vi "Glowy_Projekt.vi"() -> ()   [LabVIEW 2023]
uses:
  <vilib>/Utility/miscctls.llb/LVDateTimeRec.ctl
  stan.ctl
  Zmienn_globalne.vi
  Ogrod_zmienne.vi
  Rosliny_zmienne.vi
  Trawnik_zmienne.vi
panel:
  out "Wilgotnosc":dbl(slide)=50.0 scale=0.0..100.0
  out "Naslonecznienie":dbl(slide) scale=0.0..100.0
  in  "Przyspieszenie czasu":dbl(knob)=1.0 scale=1.0..2000.0
  out "Czas podlewania reczny":dbl
  out "date time rec":T1
  in  "Oproznianie":dbl(slide) scale=0.0..1.0
  in  "Intensywnosc opadow":dbl(slide) scale=0.0..1.0
  out "Zbiornik retencyjny":dbl(slide)=50.0 scale=0.0..100.0
  out "Aktywne podlewanie rabat roslinnych":bool
  out "Aktywne podlewanie warzywniak":bool
  out "Aktywne podlewanie sekcja 5":bool
  out "Aktywne podlewanie sekcja 4":bool
  out "Aktywne podlewanie sekcja 3":bool
  out "Aktywne podlewanie sekcja 2":bool
  out "Aktywne podlewanie sekcja 1":bool
  in  "Rosliny":bool
  in  "Ogród Warzywny":bool
  in  "Trawnik":bool
  out "Numeric":i32
  # "Trawnik"
  # "Warzywniak"
  # "DOM"
  # "Rosliny"
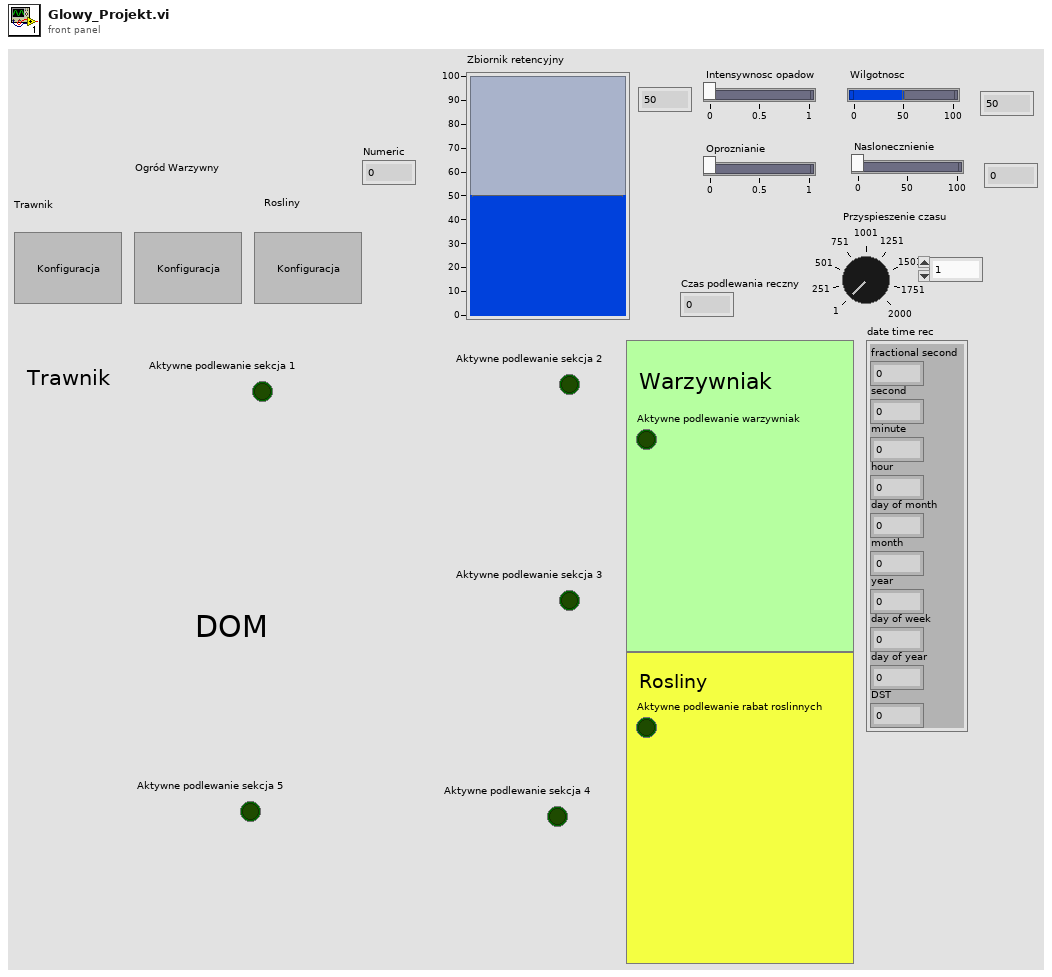
[diagram p1: front panel]
types:
  T1 = typedef "LVDateTimeRec.ctl" = cluster{"fractional second":dbl, "second":i32, "minute":i32, "hour":i32, "day of month":i32, "month":i32, "year":i32, "day of week":i32, "day of year":i32, "DST":i32}
  T2 = cluster{"Powierzchnia":i32, "Liczba zraszaczy":dbl}
  T3 = typedef "stan.ctl" = enum16{"INIT", "IDLE", "PROCESS", "EXIT"}
  T4 = enum32{"Invalid", "Standard", "Closed", "Hidden", "Minimized", "Maximized"}
  T5 = enum32{"Bad", "Idle", "Run top level", "Running"}
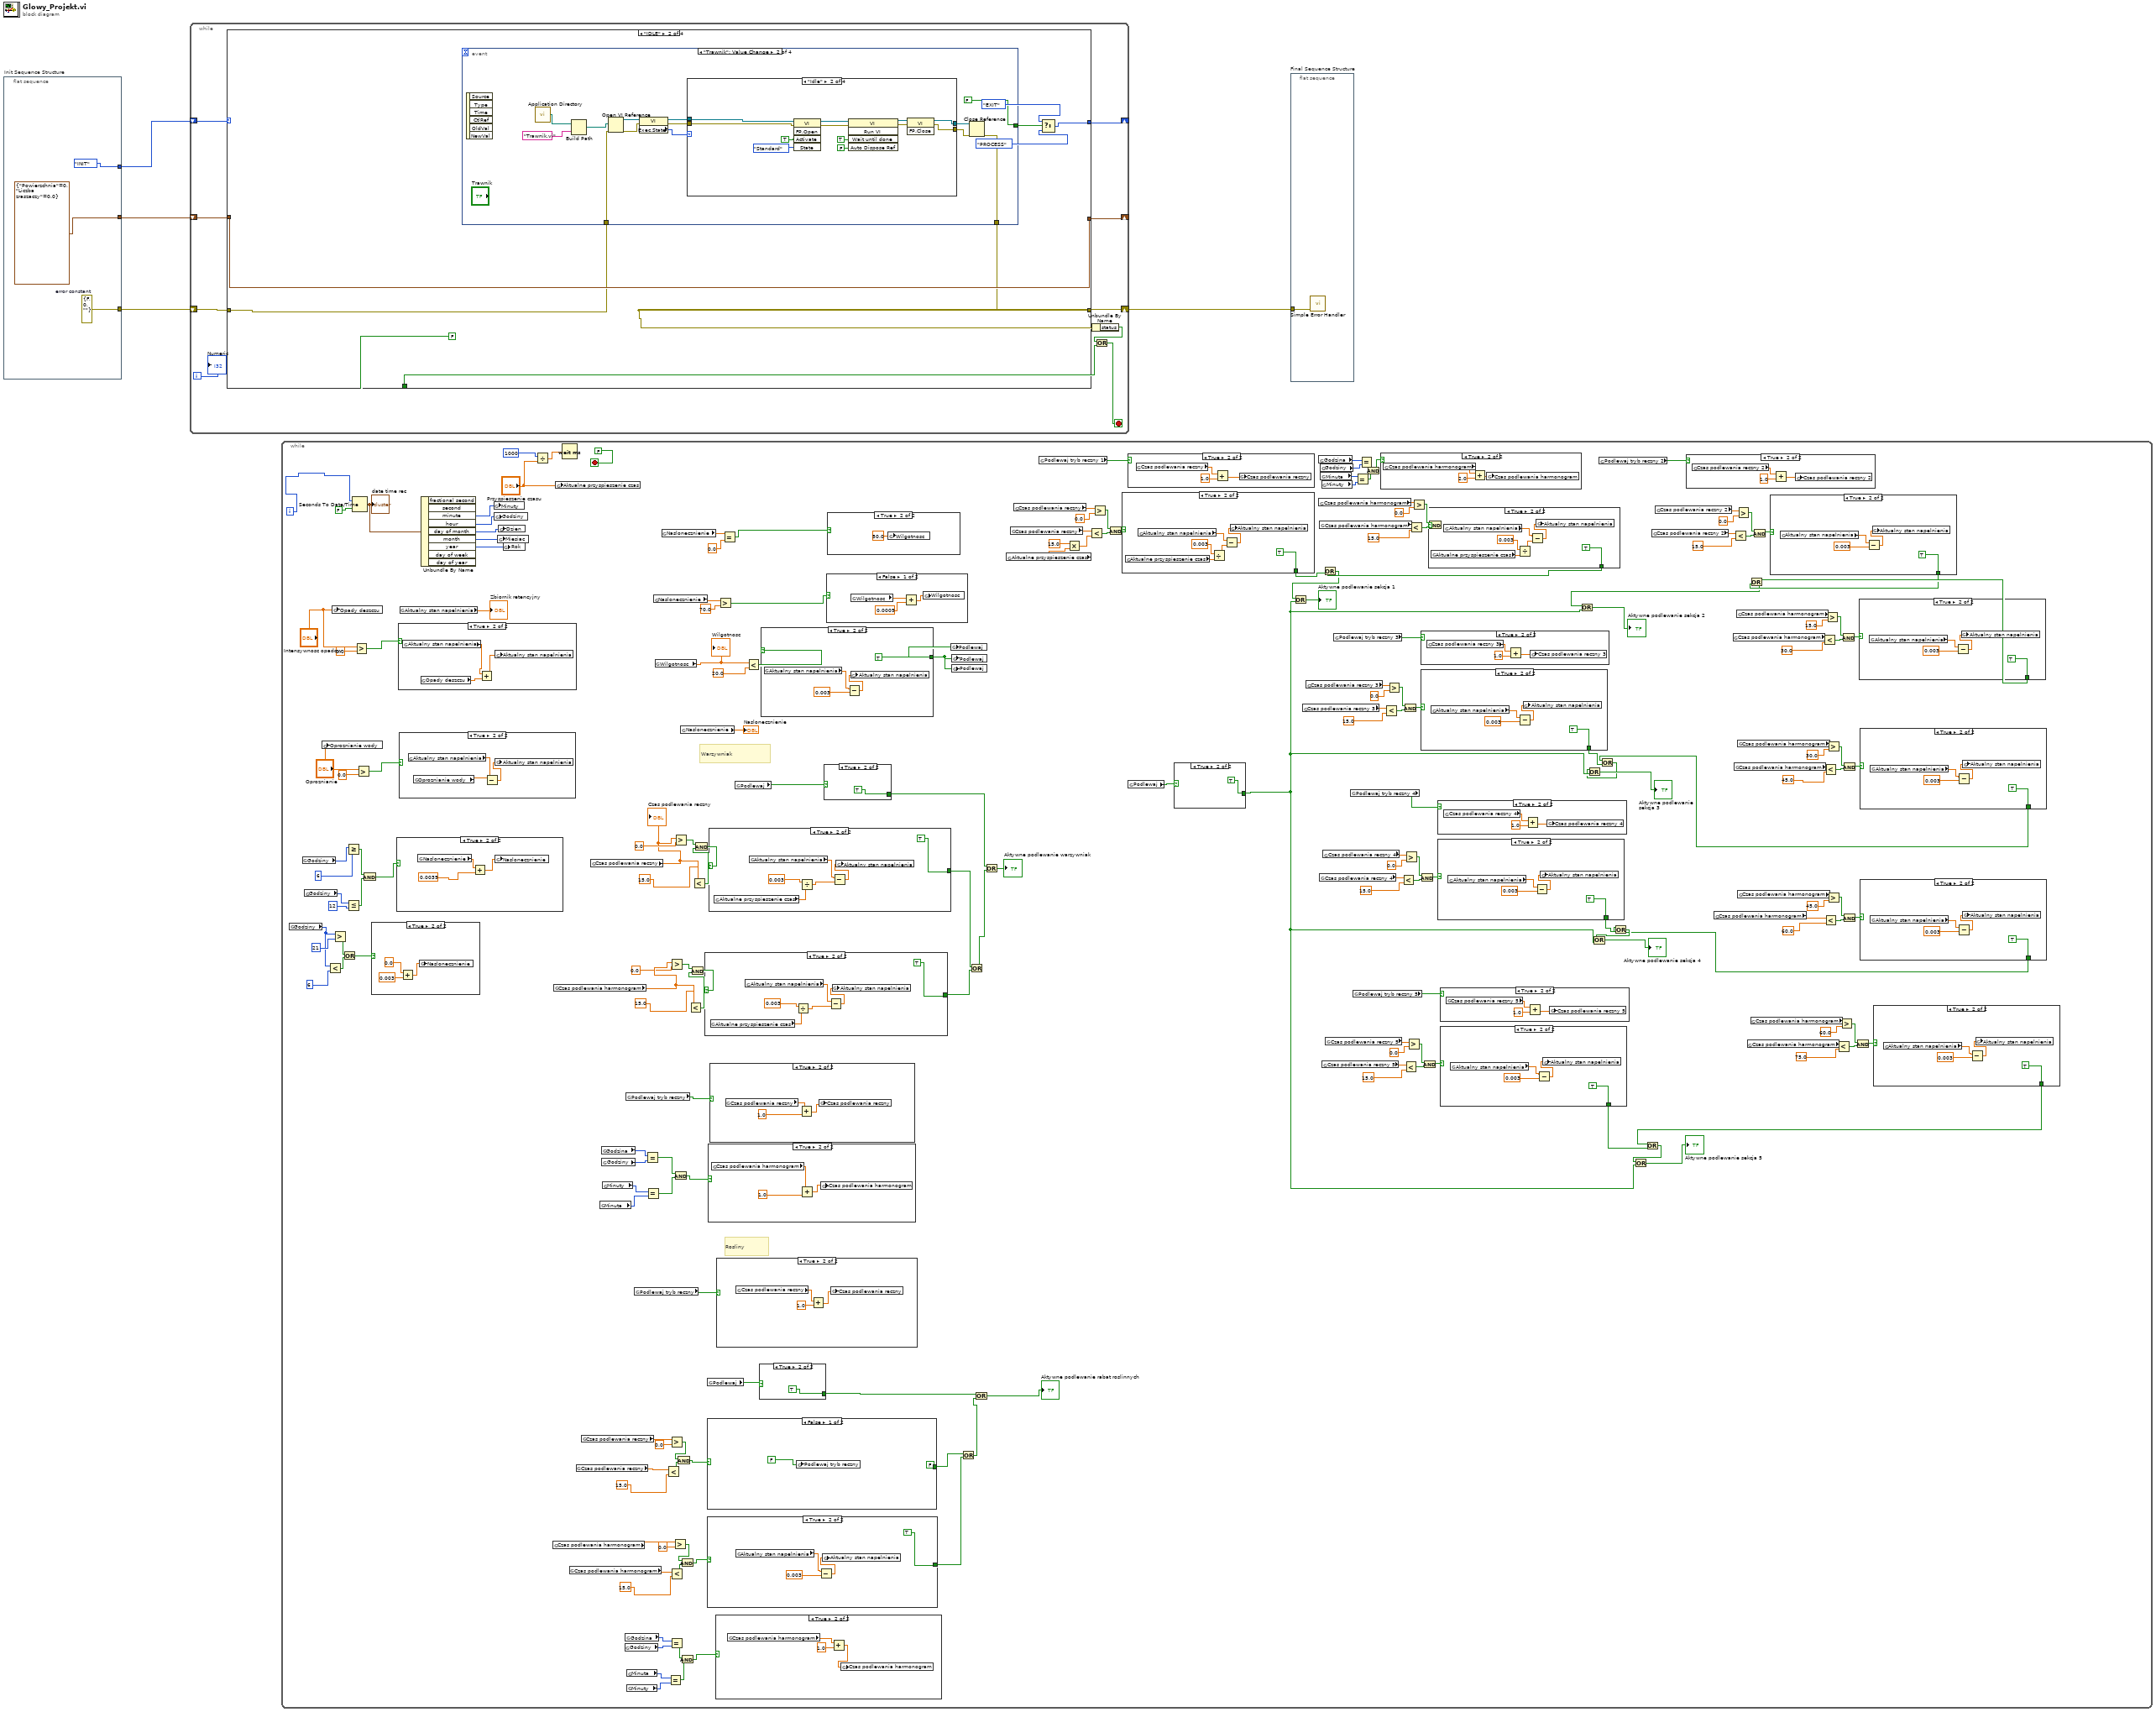
[diagram p0: block diagram]
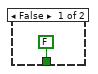
[diagram p2: hidden frame]
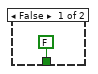
[diagram p3: hidden frame]
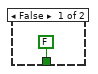
[diagram p4: hidden frame]
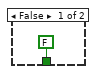
[diagram p5: hidden frame]
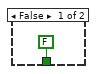
[diagram p6: hidden frame]
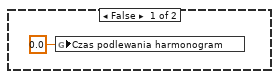
[diagram p7: hidden frame]
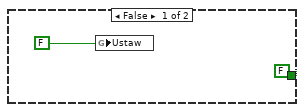
[diagram p8: hidden frame]
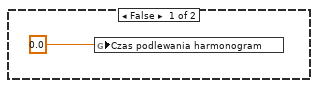
[diagram p9: hidden frame]
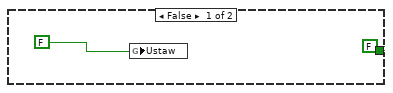
[diagram p10: hidden frame]
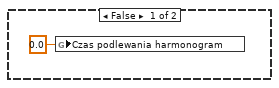
[diagram p11: hidden frame]
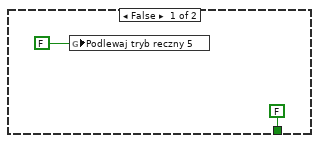
[diagram p12: hidden frame]
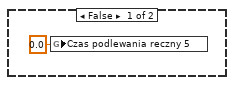
[diagram p13: hidden frame]
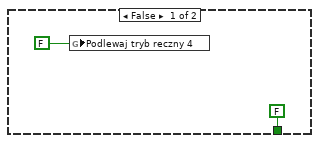
[diagram p14: hidden frame]
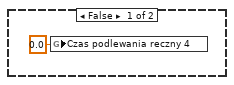
[diagram p15: hidden frame]
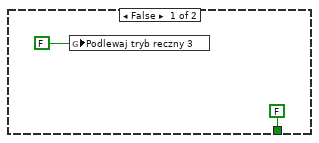
[diagram p16: hidden frame]
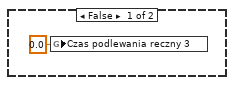
[diagram p17: hidden frame]
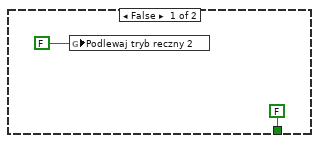
[diagram p18: hidden frame]
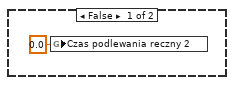
[diagram p19: hidden frame]
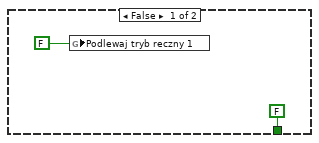
[diagram p20: hidden frame]
diagram:
  n1 = flat-sequence "Init Sequence Structure" {
    tunnel: [stan."INIT"] -> w4
    tunnel: [w6] -> w3
    tunnel: [T2 {"Powierzchnia"=0, "Liczba zraszaczy"=0.0}] -> w1
    frame #0 {
      w6 = errorcluster {"status"=FALSE, "code"=0, "source"=""}  # error constant
    }
  }
  n2 = while {
    shift-right: [w16] -> _
    shift-left: w4 -> [w17]
    shift-right: [w14] -> w2
    shift-left: w3 -> [w15]
    shift-right: [w10] -> _
    shift-left: w1 -> [w11]
    i -> [w8]
    stop <- w9 stop-if-true
    n3 = case shown="\"IDLE\"" w17 {
      tunnel: [stan."IDLE" w27 stan."IDLE" stan."EXIT"] -> w16
      tunnel: w15 -> [w18 w23 w126 w130]
      tunnel: [w18 w22 w126 w130] -> w14
      tunnel: [FALSE FALSE FALSE TRUE] -> w12
      tunnel: w11 -> [w19 w28 w125 w129]
      tunnel: [w19 w28 w125 w129] -> w10
      frame "INIT", Default {
      }
      frame "IDLE" {
        n4 = event shown="[1] \"Trawnik\": Value Change" {
          selector: _ -> [_ _ _ _]
          dyn-events: _ -> [_ _ _ _]
          timeout: _ -> [_ _ _ _]
          tunnel: [FALSE FALSE FALSE FALSE] -> w24
          tunnel: w23 -> [w30 w35 w66 w95]
          tunnel: [w30 w34 w65 w94] -> w22
          event Timeout {
            n5 = event-data() -> ()  [unwired: 1 in, 3 out]
          }
          event "Trawnik": Value Change {
            n6 = event-data() -> ()  [unwired: 1 in, 6 out]
            n7 = call <vilib>:"Application Directory.vi"() -> ("Application Directory"=w43:path)
            n8 = Build Path(base path=w43, name or relative path="Trawnik.vi") -> (appended path=w41:path)
            n9 = Open VI Reference(vi path=w41, error in (no error)=w35) -> (vi reference=w39:refnum<vi>, error out=w40:errorcluster)  [unwired: 4 in]
            n10 = property class="VI"(reference=w39, error in=w40) -> (reference out=w36:refnum<vi>, error out=w38:errorcluster, "Exec.State"=w37:T5)
            n11 = case shown="\"Idle\"" w37 {
              tunnel: [w46 w50 w60 w62] -> w33
              tunnel: w38 -> [w46 w52 w60 w62]
              tunnel: w36 -> [w45 w51 w59 w61]
              tunnel: [w45 w47 w59 w61] -> w32
              frame "Bad", Default {
              }
              frame "Idle" {
                n12 = invoke class="VI" method="FP.Open"(reference=w51, error in=w52, "Activate"=TRUE ("Activate?"), "State"=T4."Standard") -> (reference out=w56:refnum<vi>, error out=w55:errorcluster)  [unwired: 1 in, 3 out]
                n13 = invoke class="VI" method="Run VI"(reference=w56, error in=w55, "Wait until done"=TRUE ("Wait Until Done"), "Auto Dispose Ref"=FALSE ("Auto Dispose Reference")) -> (reference out=w48:refnum<vi>, error out=w49:errorcluster)  [unwired: 1 in, 3 out]
                n14 = invoke class="VI" method="FP.Close"(reference=w48, error in=w49) -> (reference out=w47:refnum<vi>, error out=w50:errorcluster)  [unwired: 1 in, 1 out]
              }
              frame "Run top level" {
              }
              frame "Running" {
              }
            }
            n15 = Close Reference(reference=w32, error in (no error)=w33) -> (error out=w34:errorcluster)
          }
          event "Ogród Warzywny": Value Change {
            n16 = event-data() -> ()  [unwired: 1 in, 6 out]
            n17 = call <vilib>:"Application Directory.vi"() -> ("Application Directory"=w74:path)
            n18 = Build Path(base path=w74, name or relative path="Ogrod_warzywny.vi") -> (appended path=w72:path)
            n19 = Open VI Reference(vi path=w72, error in (no error)=w66) -> (vi reference=w70:refnum<vi>, error out=w71:errorcluster)  [unwired: 4 in]
            n20 = property class="VI"(reference=w70, error in=w71) -> (reference out=w67:refnum<vi>, error out=w69:errorcluster, "Exec.State"=w68:T5)
            n21 = case shown="\"Idle\"" w68 {
              tunnel: [w77 w81 w91 w93] -> w64
              tunnel: w69 -> [w77 w83 w91 w93]
              tunnel: w67 -> [w76 w82 w90 w92]
              tunnel: [w76 w80 w90 w92] -> w63
              frame "Bad", Default {
              }
              frame "Idle" {
                n22 = invoke class="VI" method="FP.Open"(reference=w82, error in=w83, "Activate"=TRUE ("Activate?"), "State"=T4."Standard") -> (reference out=w87:refnum<vi>, error out=w86:errorcluster)  [unwired: 1 in, 3 out]
                n23 = invoke class="VI" method="Run VI"(reference=w87, error in=w86, "Wait until done"=TRUE ("Wait Until Done"), "Auto Dispose Ref"=FALSE ("Auto Dispose Reference")) -> (reference out=w79:refnum<vi>, error out=w78:errorcluster)  [unwired: 1 in, 3 out]
                n24 = invoke class="VI" method="FP.Close"(reference=w79, error in=w78) -> (reference out=w80:refnum<vi>, error out=w81:errorcluster)  [unwired: 1 in, 1 out]
              }
              frame "Run top level" {
              }
              frame "Running" {
              }
            }
            n25 = Close Reference(reference=w63, error in (no error)=w64) -> (error out=w65:errorcluster)
          }
          event "Rosliny": Value Change {
            n26 = event-data() -> ()  [unwired: 1 in, 6 out]
            n27 = call <vilib>:"Application Directory.vi"() -> ("Application Directory"=w105:path)
            n28 = Build Path(base path=w105, name or relative path="Rosliny.vi") -> (appended path=w103:path)
            n29 = Open VI Reference(vi path=w103, error in (no error)=w95) -> (vi reference=w101:refnum<vi>, error out=w102:errorcluster)  [unwired: 4 in]
            n30 = property class="VI"(reference=w101, error in=w102) -> (reference out=w96:refnum<vi>, error out=w98:errorcluster, "Exec.State"=w97:T5)
            n31 = case shown="\"Idle\"" w97 {
              tunnel: [w108 w110 w122 w124] -> w100
              tunnel: [w107 w109 w121 w123] -> w99
              tunnel: w98 -> [w107 w114 w121 w123]
              tunnel: w96 -> [w108 w113 w122 w124]
              frame "Bad", Default {
              }
              frame "Idle" {
                n32 = invoke class="VI" method="FP.Open"(reference=w113, error in=w114, "Activate"=TRUE ("Activate?"), "State"=T4."Standard") -> (reference out=w118:refnum<vi>, error out=w117:errorcluster)  [unwired: 1 in, 3 out]
                n33 = invoke class="VI" method="Run VI"(reference=w118, error in=w117, "Wait until done"=TRUE ("Wait Until Done"), "Auto Dispose Ref"=FALSE ("Auto Dispose Reference")) -> (reference out=w112:refnum<vi>, error out=w111:errorcluster)  [unwired: 1 in, 3 out]
                n34 = invoke class="VI" method="FP.Close"(reference=w112, error in=w111) -> (reference out=w110:refnum<vi>, error out=w109:errorcluster)  [unwired: 1 in, 1 out]
              }
              frame "Run top level" {
              }
              frame "Running" {
              }
            }
            n35 = Close Reference(reference=w100, error in (no error)=w99) -> (error out=w94:errorcluster)
          }
        }
        n36 = Select(t=stan."EXIT", s=w24, f=stan."PROCESS") -> (s? t:f=w27:T3)
      }
      frame "PROCESS" {
      }
      frame "EXIT" {
      }
    }
    n37 = Unbundle By Name(w14) -> ("status"=w13:bool)
    n38 = Or(x=w13, y=w12) -> (x .or. y?=w9:bool)
    "Numeric" <- w8
  }
  n39 = while {
    i -> [w304]
    stop <- FALSE stop-if-true
    # "Warzywniak"
    # "Rosliny"
    n40 = global read "Zmienn_globalne.vi" "Godziny"() -> (w298:i32)
    n41 = global read "Zmienn_globalne.vi" "Godziny"() -> (w294:i32)
    n42 = global read "Zmienn_globalne.vi" "Godziny"() -> (w296:i32)
    n43 = global write "Zmienn_globalne.vi" "Oproznianie wody"("Oproznianie") -> ()
    n44 = Less?(x=w298, y=6) -> (x < y?=w300:bool)
    n45 = global write "Zmienn_globalne.vi" "Opady deszczu"("Intensywnosc opadow") -> ()
    n46 = Greater?(x=w298, y=21) -> (0:w301:bool)
    n47 = Or(x=w301, y=w300) -> (x .or. y?=w302:bool)
    n48 = Greater Or Equal?(x=w294, y=6) -> (x >= y?=w292:bool)
    n49 = Less Or Equal?(x=w296, y=12) -> (x <= y?=w297:bool)
    n50 = Seconds To Date/Time(time stamp (now)=w304, to UTC (F)=FALSE) -> (date time rec=w334:T1)
    "date time rec" <- w334
    n51 = Greater?(x="Intensywnosc opadow", y=0.0) -> (0:w327:bool)
    n52 = Greater?(x="Oproznianie", y=0.0) -> (0:w332:bool)
    n53 = And(x=w292, y=w297) -> (x .and. y?=w305:bool)
    n54 = case shown="True" w302 {
      frame False {
      }
      frame True {
        n55 = Add(x=0.0, y=0.003) -> (x+y=w463:dbl)
        n56 = global write "Zmienn_globalne.vi" "Naslonecznienie"(w463) -> ()
      }
    }
    n57 = case shown="True" w305 {
      frame False {
        n58 = global read "Zmienn_globalne.vi" "Naslonecznienie"() -> (w466:dbl)
        n59 = Subtract(x=w466, y=0.003 ("x")) -> (x-y=w467:dbl)
        n60 = global write "Zmienn_globalne.vi" "Naslonecznienie"(w467) -> ()
      }
      frame True {
        n61 = global read "Zmienn_globalne.vi" "Naslonecznienie"() -> (w469:dbl)
        n62 = Add(x=w469, y=0.0039 ("x")) -> (x+y=w470:dbl)
        n63 = global write "Zmienn_globalne.vi" "Naslonecznienie"(w470) -> ()
      }
    }
    n64 = case shown="True" w327 {
      frame False {
      }
      frame True {
        n65 = global read "Zmienn_globalne.vi" "Aktualny stan napelnienia"() -> (w494:dbl)
        n66 = global read "Zmienn_globalne.vi" "Opady deszczu"() -> (w495:dbl)
        n67 = Add(x=w494, y=w495) -> (x+y=w493:dbl)
        n68 = global write "Zmienn_globalne.vi" "Aktualny stan napelnienia"(w493) -> ()
      }
    }
    n69 = case shown="True" w332 {
      frame False {
      }
      frame True {
        n70 = global read "Zmienn_globalne.vi" "Aktualny stan napelnienia"() -> (w491:dbl)
        n71 = global read "Zmienn_globalne.vi" "Oproznianie wody"() -> (w492:dbl)
        n72 = Subtract(x=w492, y=w491) -> (x-y=w490:dbl)
        n73 = global write "Zmienn_globalne.vi" "Aktualny stan napelnienia"(w490) -> ()
      }
    }
    n74 = global read "Zmienn_globalne.vi" "Aktualny stan napelnienia"() -> (→"Zbiornik retencyjny":dbl)
    n75 = Unbundle By Name(w334) -> ("minute"=w311:i32, "hour"=w312:i32, "day of month"=w326:i32, "month"=w325:i32, "year"=w324:i32)  [unwired: 4 out]
    n76 = global write "Zmienn_globalne.vi" "Minuty"(w311) -> ()
    n77 = global write "Zmienn_globalne.vi" "Godziny"(w312) -> ()
    n78 = global write "Zmienn_globalne.vi" "Miesiac"(w325) -> ()
    n79 = global write "Zmienn_globalne.vi" "Dzien"(w326) -> ()
    n80 = global write "Zmienn_globalne.vi" "Rok"(w324) -> ()
    n81 = Divide(x=u32 1000 ("milliseconds to wait"), y="Przyspieszenie czasu") -> (x/y=w309:dbl)
    n82 = global read "Rosliny_zmienne.vi" "Czas podlewania harmonogram"() -> (w217:dbl)
    n83 = global read "Ogrod_zmienne.vi" "Czas podlewania harmonogram"() -> (w205:dbl)
    n84 = global write "Zmienn_globalne.vi" "Aktualne przyspieszenie czas"("Przyspieszenie czasu") -> ()
    n85 = Wait (ms)(milliseconds to wait=w309) -> ()  [unwired: 1 out]
    n86 = global read "Rosliny_zmienne.vi" "Czas podlewania harmonogram"() -> (w219:dbl)
    n87 = global read "Rosliny_zmienne.vi" "Czas podlewania reczny"() -> (w278:dbl)
    n88 = global read "Rosliny_zmienne.vi" "Czas podlewania reczny"() -> (w280:dbl)
    n89 = global read "Ogrod_zmienne.vi" "Czas podlewania reczny"() -> (w318:dbl)
    "Czas podlewania reczny" <- w318
    n90 = global read "Ogrod_zmienne.vi" "Minuta"() -> (w211:i32)
    n91 = global read "Ogrod_zmienne.vi" "Godzina"() -> (w210:i32)
    n92 = global read "Zmienn_globalne.vi" "Godziny"() -> (w209:i32)
    n93 = global read "Zmienn_globalne.vi" "Minuty"() -> (w212:i32)
    n94 = global read "Zmienn_globalne.vi" "Godziny"() -> (w227:i32)
    n95 = global read "Rosliny_zmienne.vi" "Godzina"() -> (w228:i32)
    n96 = global read "Ogrod_zmienne.vi" "Podlewaj tryb reczny"() -> (w323:bool)
    n97 = global read "Rosliny_zmienne.vi" "Minuta"() -> (w226:i32)
    n98 = global read "Zmienn_globalne.vi" "Minuty"() -> (w225:i32)
    n99 = global read "Rosliny_zmienne.vi" "Podlewaj tryb reczny"() -> (w281:bool)
    n100 = Equal?(x=w210, y=w209) -> (x = y?=w207:bool)
    n101 = Equal?(x=w212, y=w211) -> (x = y?=w206:bool)
    n102 = global read "Zmienn_globalne.vi" "Naslonecznienie"() -> (w290:dbl)
    n103 = global read "Zmienn_globalne.vi" "Wilgotnosc"() -> (w307:dbl)
    "Wilgotnosc" <- w307
    n104 = global read "Zmienn_globalne.vi" "Naslonecznienie"() -> (w287:dbl)
    n105 = Less?(x=w278, y=15.0) -> (x < y?=w274:bool)
    n106 = Equal?(x=w226, y=w225) -> (x = y?=w223:bool)
    n107 = Greater?(x=w280, y=0.0) -> (0:w273:bool)
    n108 = Equal?(x=w228, y=w227) -> (x = y?=w224:bool)
    n109 = Greater?(x=w205, y=0.0) -> (0:w201:bool)
    n110 = Less?(x=w219, y=15.0) -> (x < y?=w221:bool)
    n111 = Greater?(x=w217, y=0.0) -> (0:w222:bool)
    n112 = Greater?(x=w318, y=0.0) -> (0:w322:bool)
    n113 = And(x=w207, y=w206) -> (x .and. y?=w208:bool)
    n114 = And(x=w273, y=w274) -> (x .and. y?=w275:bool)
    n115 = And(x=w222, y=w221) -> (x .and. y?=w220:bool)
    n116 = And(x=w224, y=w223) -> (x .and. y?=w213:bool)
    n117 = global read "Zmienn_globalne.vi" "Naslonecznienie"() -> (→"Naslonecznienie":dbl)
    n118 = Less?(x=w205, y=15.0) -> (x < y?=w203:bool)
    n119 = And(x=w201, y=w203) -> (x .and. y?=w202:bool)
    n120 = Less?(x=w318, y=15.0) -> (x < y?=w320:bool)
    n121 = And(x=w322, y=w320) -> (x .and. y?=w321:bool)
    n122 = case shown="True" w202 {
      tunnel: [FALSE TRUE] -> w198
      frame False {
        n123 = global write "Ogrod_zmienne.vi" "Ustaw"(FALSE ("Podlewaj tryb reczny")) -> ()
      }
      frame True {
        n124 = global read "Zmienn_globalne.vi" "Aktualne przyspieszenie czas"() -> (w369:dbl)
        n125 = global read "Zmienn_globalne.vi" "Aktualny stan napelnienia"() -> (w372:dbl)
        n126 = Divide(x=0.003 ("y"), y=w369) -> (x/y=w371:dbl)
        n127 = Subtract(x=w372, y=w371) -> (x-y=w373:dbl)
        n128 = global write "Zmienn_globalne.vi" "Aktualny stan napelnienia"(w373) -> ()
      }
    }
    n129 = case shown="False" w275 {
      tunnel: [FALSE TRUE] -> w216
      frame False {
        n130 = global write "Rosliny_zmienne.vi" "Podlewaj tryb reczny"(FALSE ("Podlewaj tryb reczny")) -> ()
      }
      frame True {
        n131 = global read "Zmienn_globalne.vi" "Aktualny stan napelnienia"() -> (w444:dbl)
        n132 = Subtract(x=w444, y=0.003) -> (x-y=w445:dbl)
        n133 = global write "Zmienn_globalne.vi" "Aktualny stan napelnienia"(w445) -> ()
      }
    }
    n134 = global read "Rosliny_zmienne.vi" "Podlewaj"() -> (w282:bool)
    n135 = case shown="True" w220 {
      tunnel: [FALSE TRUE] -> w215
      frame False {
        n136 = global write "Rosliny_zmienne.vi" "Ustaw"(FALSE ("Podlewaj tryb reczny")) -> ()
      }
      frame True {
        n137 = global read "Zmienn_globalne.vi" "Aktualny stan napelnienia"() -> (w382:dbl)
        n138 = Subtract(x=w382, y=0.003) -> (x-y=w383:dbl)
        n139 = global write "Zmienn_globalne.vi" "Aktualny stan napelnienia"(w383) -> ()
      }
    }
    n140 = case shown="True" w208 {
      frame False {
        n141 = global write "Ogrod_zmienne.vi" "Czas podlewania harmonogram"(0.0 ("Czas podlewania reczny")) -> ()
      }
      frame True {
        n142 = global read "Ogrod_zmienne.vi" "Czas podlewania harmonogram"() -> (w377:dbl)
        n143 = Add(x=w377, y=1.0) -> (x+y=w378:dbl)
        n144 = global write "Ogrod_zmienne.vi" "Czas podlewania harmonogram"(w378) -> ()
      }
    }
    n145 = case shown="True" w321 {
      tunnel: [FALSE TRUE] -> w199
      frame False {
        n146 = global write "Ogrod_zmienne.vi" "Podlewaj tryb reczny"(FALSE ("Podlewaj tryb reczny")) -> ()
      }
      frame True {
        n147 = global read "Zmienn_globalne.vi" "Aktualne przyspieszenie czas"() -> (w480:dbl)
        n148 = global read "Zmienn_globalne.vi" "Aktualny stan napelnienia"() -> (w483:dbl)
        n149 = Divide(x=0.003 ("y"), y=w480) -> (x/y=w482:dbl)
        n150 = Subtract(x=w483, y=w482) -> (x-y=w484:dbl)
        n151 = global write "Zmienn_globalne.vi" "Aktualny stan napelnienia"(w484) -> ()
      }
    }
    n152 = case shown="True" w323 {
      frame False {
        n153 = global write "Ogrod_zmienne.vi" "Czas podlewania reczny"(0.0 ("Czas podlewania reczny")) -> ()
      }
      frame True {
        n154 = global read "Ogrod_zmienne.vi" "Czas podlewania reczny"() -> (w488:dbl)
        n155 = Add(x=w488, y=1.0) -> (x+y=w489:dbl)
        n156 = global write "Ogrod_zmienne.vi" "Czas podlewania reczny"(w489) -> ()
      }
    }
    n157 = case shown="True" w213 {
      frame False {
        n158 = global write "Rosliny_zmienne.vi" "Czas podlewania harmonogram"(0.0 ("Czas podlewania harmonogram")) -> ()
      }
      frame True {
        n159 = global read "Rosliny_zmienne.vi" "Czas podlewania harmonogram"() -> (w388:dbl)
        n160 = Add(x=w388, y=1.0) -> (x+y=w386:dbl)
        n161 = global write "Rosliny_zmienne.vi" "Czas podlewania harmonogram"(w386) -> ()
      }
    }
    n162 = case shown="True" w281 {
      frame False {
        n163 = global write "Rosliny_zmienne.vi" "Czas podlewania reczny"(0.0 ("Czas podlewania reczny")) -> ()
      }
      frame True {
        n164 = global read "Rosliny_zmienne.vi" "Czas podlewania reczny"() -> (w449:dbl)
        n165 = Add(x=w449, y=1.0) -> (x+y=w450:dbl)
        n166 = global write "Rosliny_zmienne.vi" "Czas podlewania reczny"(w450) -> ()
      }
    }
    n167 = Greater?(x=w290, y=70.0) -> (0:w288:bool)
    n168 = Equal?(x=w287, y=0.0) -> (x = y?=w285:bool)
    n169 = global read "Ogrod_zmienne.vi" "Podlewaj"() -> (w316:bool)
    n170 = Less?(x=w307, y=20.0) -> (x < y?=w291:bool)
    n171 = case shown="True" w282 {
      tunnel: [FALSE TRUE] -> w276
      frame False {
      }
      frame True {
      }
    }
    n172 = case shown="True" w291 {
      tunnel: [FALSE TRUE] -> w284
      frame False {
      }
      frame True {
        n173 = global read "Zmienn_globalne.vi" "Aktualny stan napelnienia"() -> (w476:dbl)
        n174 = Subtract(x=w476, y=0.003) -> (x-y=w475:dbl)
        n175 = global write "Zmienn_globalne.vi" "Aktualny stan napelnienia"(w475) -> ()
      }
    }
    n176 = case shown="True" w316 {
      tunnel: [FALSE TRUE] -> w315
      frame False {
      }
      frame True {
      }
    }
    n177 = case shown="False" w288 {
      frame False {
        n178 = global read "Zmienn_globalne.vi" "Wilgotnosc"() -> (w457:dbl)
        n179 = Add(x=w457, y=0.0009) -> (x+y=w458:dbl)
        n180 = global write "Zmienn_globalne.vi" "Wilgotnosc"(w458) -> ()
      }
      frame True {
        n181 = global read "Zmienn_globalne.vi" "Wilgotnosc"() -> (w460:dbl)
        n182 = Subtract(x=w460, y=0.0029) -> (x-y=w461:dbl)
        n183 = global write "Zmienn_globalne.vi" "Wilgotnosc"(w461) -> ()
      }
    }
    n184 = case shown="True" w285 {
      frame False {
      }
      frame True {
        n185 = global write "Zmienn_globalne.vi" "Wilgotnosc"(50.0 ("Wilgotnosc")) -> ()
      }
    }
    n186 = global write "Ogrod_zmienne.vi" "Podlewaj"(w284) -> ()
    n187 = global write "Trawnik_zmienne.vi" "Podlewaj"(w284) -> ()
    n188 = global write "Rosliny_zmienne.vi" "Podlewaj"(w284) -> ()
    n189 = Or(x=w216, y=w215) -> (x .or. y?=w214:bool)
    n190 = Or(x=w199, y=w198) -> (x .or. y?=w200:bool)
    n191 = Or(x=w276, y=w214) -> (x .or. y?=→"Aktywne podlewanie rabat roslinnych":bool)
    n192 = Or(x=w315, y=w200) -> (x .or. y?=→"Aktywne podlewanie warzywniak":bool)
    n193 = global read "Zmienn_globalne.vi" "Aktualne przyspieszenie czas"() -> (w268:dbl)
    n194 = global read "Trawnik_zmienne.vi" "Czas podlewania reczny"() -> (w270:dbl)
    n195 = global read "Trawnik_zmienne.vi" "Czas podlewania reczny"() -> (w272:dbl)
    n196 = global read "Trawnik_zmienne.vi" "Podlewaj tryb reczny 1"() -> (w262:bool)
    n197 = Multiply(x=15.0, y=w268) -> (x*y=w267:dbl)
    n198 = Less?(x=w270, y=w267) -> (x < y?=w265:bool)
    n199 = Greater?(x=w272, y=0.0) -> (0:w266:bool)
    n200 = And(x=w266, y=w265) -> (x .and. y?=w264:bool)
    n201 = case shown="True" w264 {
      tunnel: [FALSE TRUE] -> w183
      frame False {
        n202 = global write "Trawnik_zmienne.vi" "Podlewaj tryb reczny 1"(FALSE ("Podlewaj tryb reczny")) -> ()
      }
      frame True {
        n203 = global read "Zmienn_globalne.vi" "Aktualne przyspieszenie czas"() -> (w431:dbl)
        n204 = global read "Zmienn_globalne.vi" "Aktualny stan napelnienia"() -> (w436:dbl)
        n205 = Divide(x=0.003 ("y"), y=w431) -> (x/y=w433:dbl)
        n206 = Subtract(x=w436, y=w433) -> (x-y=w435:dbl)
        n207 = global write "Zmienn_globalne.vi" "Aktualny stan napelnienia"(w435) -> ()
      }
    }
    n208 = case shown="True" w262 {
      frame False {
        n209 = global write "Trawnik_zmienne.vi" "Czas podlewania reczny"(0.0 ("Czas podlewania reczny")) -> ()
      }
      frame True {
        n210 = global read "Trawnik_zmienne.vi" "Czas podlewania reczny"() -> (w440:dbl)
        n211 = Add(x=w440, y=1.0) -> (x+y=w438:dbl)
        n212 = global write "Trawnik_zmienne.vi" "Czas podlewania reczny"(w438) -> ()
      }
    }
    n213 = global read "Trawnik_zmienne.vi" "Podlewaj"() -> (w283:bool)
    n214 = case shown="True" w283 {
      tunnel: [FALSE TRUE] -> w229
      frame False {
      }
      frame True {
      }
    }
    n215 = global read "Trawnik_zmienne.vi" "Czas podlewania reczny 3"() -> (w251:dbl)
    n216 = global read "Trawnik_zmienne.vi" "Czas podlewania reczny 3"() -> (w253:dbl)
    n217 = global read "Trawnik_zmienne.vi" "Godzina"() -> (w197:i32)
    n218 = global read "Trawnik_zmienne.vi" "Czas podlewania harmonogram"() -> (w185:dbl)
    n219 = global read "Trawnik_zmienne.vi" "Czas podlewania harmonogram"() -> (w187:dbl)
    n220 = global read "Trawnik_zmienne.vi" "Czas podlewania reczny 4"() -> (w243:dbl)
    n221 = global read "Zmienn_globalne.vi" "Godziny"() -> (w196:i32)
    n222 = global read "Trawnik_zmienne.vi" "Minuta"() -> (w195:i32)
    n223 = global read "Zmienn_globalne.vi" "Minuty"() -> (w194:i32)
    n224 = global read "Trawnik_zmienne.vi" "Czas podlewania reczny 5"() -> (w233:dbl)
    n225 = global read "Trawnik_zmienne.vi" "Czas podlewania reczny 4"() -> (w245:dbl)
    n226 = global read "Trawnik_zmienne.vi" "Czas podlewania reczny 5"() -> (w231:dbl)
    n227 = global read "Trawnik_zmienne.vi" "Podlewaj tryb reczny 3"() -> (w247:bool)
    n228 = global read "Trawnik_zmienne.vi" "Podlewaj tryb reczny 4"() -> (w239:bool)
    n229 = global read "Trawnik_zmienne.vi" "Podlewaj tryb reczny 5"() -> (w237:bool)
    n230 = Equal?(x=w195, y=w194) -> (x = y?=w191:bool)
    n231 = Equal?(x=w197, y=w196) -> (x = y?=w192:bool)
    n232 = And(x=w192, y=w191) -> (x .and. y?=w193:bool)
    n233 = case shown="True" w193 {
      frame False {
        n234 = global write "Trawnik_zmienne.vi" "Czas podlewania harmonogram"(0.0 ("Czas podlewania harmonogram")) -> ()
      }
      frame True {
        n235 = global read "Trawnik_zmienne.vi" "Czas podlewania harmonogram"() -> (w366:dbl)
        n236 = Add(x=w366, y=2.0) -> (x+y=w364:dbl)
        n237 = global write "Trawnik_zmienne.vi" "Czas podlewania harmonogram"(w364) -> ()
      }
    }
    n238 = Less?(x=w251, y=15.0 ("x")) -> (x < y?=w249:bool)
    n239 = Greater?(x=w253, y=0.0) -> (0:w250:bool)
    n240 = Less?(x=w243, y=15.0 ("x")) -> (x < y?=w241:bool)
    n241 = And(x=w250, y=w249) -> (x .and. y?=w248:bool)
    n242 = Less?(x=w233, y=15.0 ("x")) -> (x < y?=w235:bool)
    n243 = Greater?(x=w245, y=0.0) -> (0:w242:bool)
    n244 = Greater?(x=w231, y=0.0) -> (0:w234:bool)
    n245 = Less?(x=w187, y=15.0 ("x")) -> (x < y?=w189:bool)
    n246 = Greater?(x=w185, y=0.0) -> (0:w188:bool)
    n247 = And(x=w242, y=w241) -> (x .and. y?=w240:bool)
    n248 = case shown="True" w247 {
      frame False {
        n249 = global write "Trawnik_zmienne.vi" "Czas podlewania reczny 3"(0.0 ("Czas podlewania reczny")) -> ()
      }
      frame True {
        n250 = global read "Trawnik_zmienne.vi" "Czas podlewania reczny 3"() -> (w418:dbl)
        n251 = Add(x=w418, y=1.0) -> (x+y=w416:dbl)
        n252 = global write "Trawnik_zmienne.vi" "Czas podlewania reczny 3"(w416) -> ()
      }
    }
    n253 = case shown="True" w248 {
      tunnel: [FALSE TRUE] -> w165
      frame False {
        n254 = global write "Trawnik_zmienne.vi" "Podlewaj tryb reczny 3"(FALSE ("Podlewaj tryb reczny")) -> ()
      }
      frame True {
        n255 = global read "Zmienn_globalne.vi" "Aktualny stan napelnienia"() -> (w413:dbl)
        n256 = Subtract(x=w413, y=0.003) -> (x-y=w412:dbl)
        n257 = global write "Zmienn_globalne.vi" "Aktualny stan napelnienia"(w412) -> ()
      }
    }
    n258 = And(x=w234, y=w235) -> (x .and. y?=w236:bool)
    n259 = And(x=w188, y=w189) -> (x .and. y?=w190:bool)
    n260 = case shown="True" w190 {
      tunnel: [FALSE TRUE] -> w184
      frame False {
      }
      frame True {
        n261 = global read "Zmienn_globalne.vi" "Aktualne przyspieszenie czas"() -> (w357:dbl)
        n262 = global read "Zmienn_globalne.vi" "Aktualny stan napelnienia"() -> (w362:dbl)
        n263 = Divide(x=0.003 ("y"), y=w357) -> (x/y=w359:dbl)
        n264 = Subtract(x=w362, y=w359) -> (x-y=w361:dbl)
        n265 = global write "Zmienn_globalne.vi" "Aktualny stan napelnienia"(w361) -> ()
      }
    }
    n266 = Or(x=w184, y=w183) -> (x .or. y?=w182:bool)
    n267 = Or(x=w182, y=w229) -> (x .or. y?=→"Aktywne podlewanie sekcja 1":bool)
    n268 = case shown="True" w239 {
      frame False {
        n269 = global write "Trawnik_zmienne.vi" "Czas podlewania reczny 4"(0.0 ("Czas podlewania reczny")) -> ()
      }
      frame True {
        n270 = global read "Trawnik_zmienne.vi" "Czas podlewania reczny 4"() -> (w408:dbl)
        n271 = Add(x=w408, y=1.0) -> (x+y=w406:dbl)
        n272 = global write "Trawnik_zmienne.vi" "Czas podlewania reczny 4"(w406) -> ()
      }
    }
    n273 = case shown="True" w240 {
      tunnel: [FALSE TRUE] -> w157
      frame False {
        n274 = global write "Trawnik_zmienne.vi" "Podlewaj tryb reczny 4"(FALSE ("Podlewaj tryb reczny")) -> ()
      }
      frame True {
        n275 = global read "Zmienn_globalne.vi" "Aktualny stan napelnienia"() -> (w403:dbl)
        n276 = Subtract(x=w403, y=0.003) -> (x-y=w402:dbl)
        n277 = global write "Zmienn_globalne.vi" "Aktualny stan napelnienia"(w402) -> ()
      }
    }
    n278 = case shown="True" w237 {
      frame False {
        n279 = global write "Trawnik_zmienne.vi" "Czas podlewania reczny 5"(0.0 ("Czas podlewania reczny")) -> ()
      }
      frame True {
        n280 = global read "Trawnik_zmienne.vi" "Czas podlewania reczny 5"() -> (w398:dbl)
        n281 = Add(x=w398, y=1.0) -> (x+y=w396:dbl)
        n282 = global write "Trawnik_zmienne.vi" "Czas podlewania reczny 5"(w396) -> ()
      }
    }
    n283 = case shown="True" w236 {
      tunnel: [FALSE TRUE] -> w148
      frame False {
        n284 = global write "Trawnik_zmienne.vi" "Podlewaj tryb reczny 5"(FALSE ("Podlewaj tryb reczny")) -> ()
      }
      frame True {
        n285 = global read "Zmienn_globalne.vi" "Aktualny stan napelnienia"() -> (w393:dbl)
        n286 = Subtract(x=w393, y=0.003) -> (x-y=w392:dbl)
        n287 = global write "Zmienn_globalne.vi" "Aktualny stan napelnienia"(w392) -> ()
      }
    }
    n288 = global read "Trawnik_zmienne.vi" "Podlewaj tryb reczny 2"() -> (w261:bool)
    n289 = global read "Trawnik_zmienne.vi" "Czas podlewania reczny 2"() -> (w257:dbl)
    n290 = global read "Trawnik_zmienne.vi" "Czas podlewania reczny 2"() -> (w255:dbl)
    n291 = case shown="True" w261 {
      frame False {
        n292 = global write "Trawnik_zmienne.vi" "Czas podlewania reczny 2"(0.0 ("Czas podlewania reczny")) -> ()
      }
      frame True {
        n293 = global read "Trawnik_zmienne.vi" "Czas podlewania reczny 2"() -> (w428:dbl)
        n294 = Add(x=w428, y=1.0) -> (x+y=w426:dbl)
        n295 = global write "Trawnik_zmienne.vi" "Czas podlewania reczny 2"(w426) -> ()
      }
    }
    n296 = global read "Trawnik_zmienne.vi" "Czas podlewania harmonogram"() -> (w161:dbl)
    n297 = Less?(x=w257, y=15.0 ("x")) -> (x < y?=w259:bool)
    n298 = global read "Trawnik_zmienne.vi" "Czas podlewania harmonogram"() -> (w179:dbl)
    n299 = global read "Trawnik_zmienne.vi" "Czas podlewania harmonogram"() -> (w169:dbl)
    n300 = Greater?(x=w255, y=0.0) -> (0:w258:bool)
    n301 = global read "Trawnik_zmienne.vi" "Czas podlewania harmonogram"() -> (w181:dbl)
    n302 = global read "Trawnik_zmienne.vi" "Czas podlewania harmonogram"() -> (w167:dbl)
    n303 = global read "Trawnik_zmienne.vi" "Czas podlewania harmonogram"() -> (w163:dbl)
    n304 = global read "Trawnik_zmienne.vi" "Czas podlewania harmonogram"() -> (w151:dbl)
    n305 = global read "Trawnik_zmienne.vi" "Czas podlewania harmonogram"() -> (w149:dbl)
    n306 = And(x=w258, y=w259) -> (x .and. y?=w260:bool)
    n307 = case shown="True" w260 {
      tunnel: [FALSE TRUE] -> w174
      frame False {
        n308 = global write "Trawnik_zmienne.vi" "Podlewaj tryb reczny 2"(FALSE ("Podlewaj tryb reczny")) -> ()
      }
      frame True {
        n309 = global read "Zmienn_globalne.vi" "Aktualny stan napelnienia"() -> (w423:dbl)
        n310 = Subtract(x=w423, y=0.003) -> (x-y=w422:dbl)
        n311 = global write "Zmienn_globalne.vi" "Aktualny stan napelnienia"(w422) -> ()
      }
    }
    n312 = Less?(x=w179, y=30.0 ("x")) -> (x < y?=w177:bool)
    n313 = Less?(x=w169, y=45.0 ("x")) -> (x < y?=w171:bool)
    n314 = Less?(x=w161, y=60.0 ("x")) -> (x < y?=w159:bool)
    n315 = Greater?(x=w181, y=15.0) -> (0:w178:bool)
    n316 = Greater?(x=w167, y=30.0) -> (0:w170:bool)
    n317 = Greater?(x=w163, y=45.0) -> (0:w160:bool)
    n318 = Less?(x=w151, y=75.0 ("x")) -> (x < y?=w153:bool)
    n319 = Greater?(x=w149, y=60.0) -> (0:w152:bool)
    n320 = And(x=w178, y=w177) -> (x .and. y?=w176:bool)
    n321 = And(x=w170, y=w171) -> (x .and. y?=w172:bool)
    n322 = And(x=w160, y=w159) -> (x .and. y?=w158:bool)
    n323 = And(x=w152, y=w153) -> (x .and. y?=w154:bool)
    n324 = case shown="True" w176 {
      tunnel: [FALSE TRUE] -> w175
      frame False {
      }
      frame True {
        n325 = global read "Zmienn_globalne.vi" "Aktualny stan napelnienia"() -> (w354:dbl)
        n326 = Subtract(x=w354, y=0.003) -> (x-y=w353:dbl)
        n327 = global write "Zmienn_globalne.vi" "Aktualny stan napelnienia"(w353) -> ()
      }
    }
    n328 = Or(x=w175, y=w174) -> (x .or. y?=w173:bool)
    n329 = Or(x=w173, y=w229) -> (x .or. y?=→"Aktywne podlewanie sekcja 2":bool)
    n330 = case shown="True" w172 {
      tunnel: [FALSE TRUE] -> w166
      frame False {
      }
      frame True {
        n331 = global read "Zmienn_globalne.vi" "Aktualny stan napelnienia"() -> (w349:dbl)
        n332 = Subtract(x=w349, y=0.003) -> (x-y=w348:dbl)
        n333 = global write "Zmienn_globalne.vi" "Aktualny stan napelnienia"(w348) -> ()
      }
    }
    n334 = Or(x=w166, y=w165) -> (x .or. y?=w164:bool)
    n335 = Or(x=w164, y=w229) -> (x .or. y?=→"Aktywne podlewanie sekcja 3":bool)
    n336 = case shown="True" w158 {
      tunnel: [FALSE TRUE] -> w155
      frame False {
      }
      frame True {
        n337 = global read "Zmienn_globalne.vi" "Aktualny stan napelnienia"() -> (w344:dbl)
        n338 = Subtract(x=w344, y=0.003) -> (x-y=w343:dbl)
        n339 = global write "Zmienn_globalne.vi" "Aktualny stan napelnienia"(w343) -> ()
      }
    }
    n340 = Or(x=w155, y=w157) -> (x .or. y?=w156:bool)
    n341 = Or(x=w156, y=w229) -> (x .or. y?=→"Aktywne podlewanie sekcja 4":bool)
    n342 = case shown="True" w154 {
      tunnel: [FALSE TRUE] -> w146
      frame False {
      }
      frame True {
        n343 = global read "Zmienn_globalne.vi" "Aktualny stan napelnienia"() -> (w339:dbl)
        n344 = Subtract(x=w339, y=0.003) -> (x-y=w338:dbl)
        n345 = global write "Zmienn_globalne.vi" "Aktualny stan napelnienia"(w338) -> ()
      }
    }
    n346 = Or(x=w146, y=w148) -> (x .or. y?=w147:bool)
    n347 = Or(x=w147, y=w229) -> (x .or. y?=→"Aktywne podlewanie sekcja 5":bool)
  }
  n348 = flat-sequence "Final Sequence Structure" {
    tunnel: w2 -> [w496]
    frame #0 {
      n349 = call <vilib>:"Simple Error Handler.vi"("error in (no error)"=w496) -> ()  [unwired: 4 in, 5 out]
    }
  }
